vi "Get Terminal Address.vi"(8 "error in":errorcluster, 11 "port in":T1 format="%.0x") -> (0 "error out":errorcluster, 2 "port number":u16, 3 "port out":T1 format="%.0x", 4 "found?":bool)   [LabVIEW 2020, in "Ballard MIL-STD-1553 Scripting.lvlib"]
uses:
  Ballard MIL-STD-1553 Scripting.lvlib
  <vilib>/NI VeriStand/Custom Device API/Custom Device Item Ref.ctl
  Constants.vi
  <vilib>/NI VeriStand/Custom Device API/Get Item Property (U16).vi
  <vilib>/NI VeriStand/Custom Device API/Custom Device API.lvlib
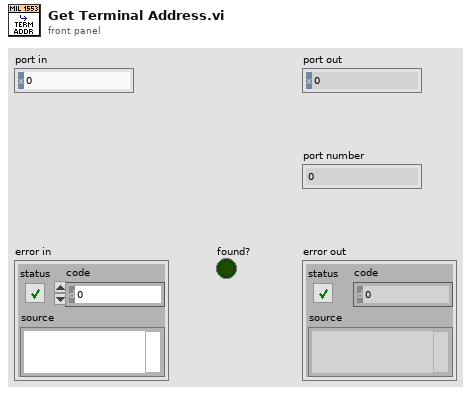
[diagram p1: front panel]
types:
  T1 = typedef "Custom Device API.lvlib/Custom Device Item Ref.ctl" = u64
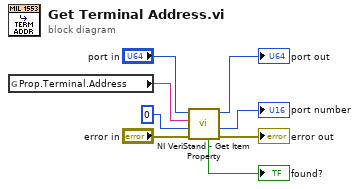
[diagram p0: block diagram]
diagram:
  n1 = global read "Constants.vi" "Prop.Terminal.Address"() -> (w3:string)
  n2 = call-poly <vilib>:"NI VeriStand - Get Item Property.vi"("error in (no error)"="error in", "Default Value"=u16 0, "Property Name"=w3, "Item Ref in"="port in") -> ("error out"=→"error out":errorcluster, "Value"=→"port number":u16, "Item Ref out"=→"port out":T1, "Found?"=→"found?":bool)  [unwired: 4 in]
